vi "Login.vi"() -> ()   [LabVIEW 2020]
uses:
  Global1.vi
panel:
  in  "联机模式":enum16{"单机", "追溯"}(ring)
  in  "密码":string
  in  "账号":string
  in  "确定":bool
  # "芯轴分总成磨合台"
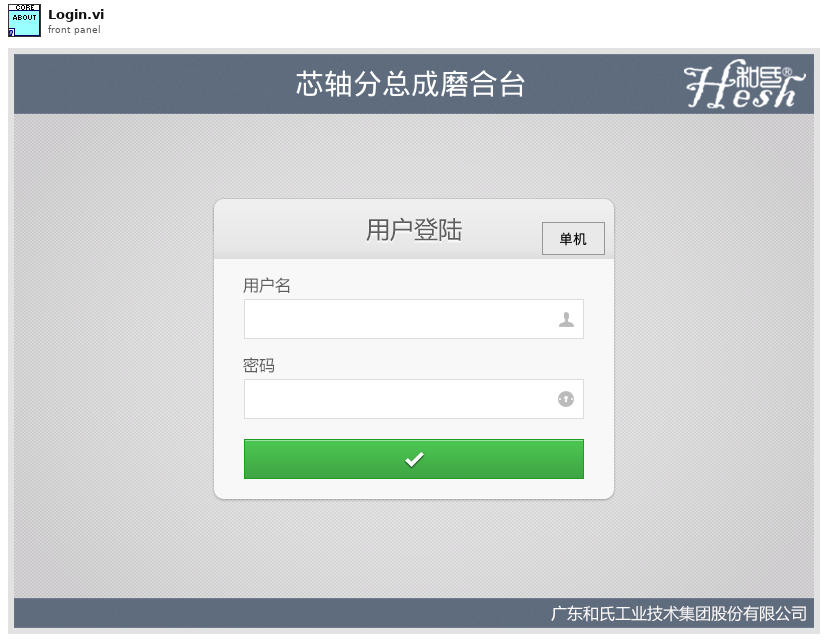
[diagram p1: front panel]
types:
  T1 = enum32{"Invalid", "Standard", "Closed", "Hidden", "Minimized", "Maximized"}
  T2 = enum8{"Enabled", "Disabled", "Disabled and Grayed Out"}
  T3 = cluster{"data[0]":string, "data[1]":string, "data[2]":string, "data[3]":string}
  T4 = typedef "eventvkey.ctl" = enum16{"ASCII", "Enter", "Return", "Shift", "Ctrl", "Alt", "Cmd", "Opt", "Caps", "NumLock", "Clear", "Break", "Up", "Down", "Left", "Right", "Insert", "Delete", "Home", "End", "PageUp", "PageDown", "Escape", "Help", "Pause", "ScrollLock", "F1", "F2", "F3", "F4", "F5", "F6", "F7", "F8", "F9", "F10", "F11", "F12", "F13", "F14", "F15", "F16", "F17", "F18", "F19", "F20", "F21", "F22", "F23", "F24", "Play", "VolumeUp", "VolumeDown", "Mute", "Two Byte Char"}
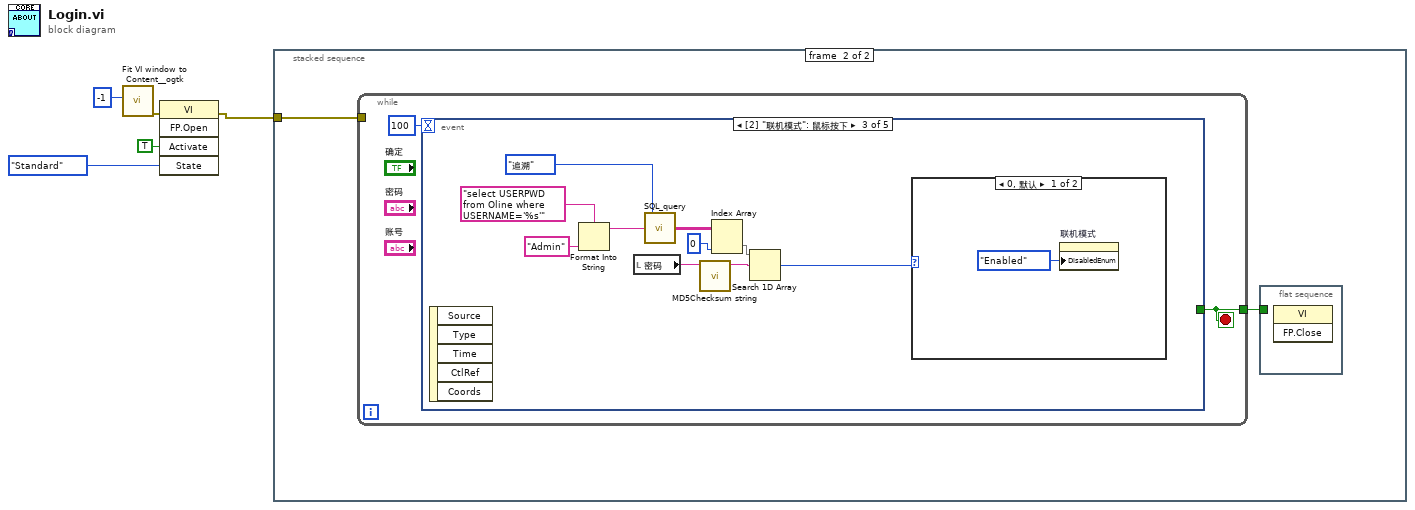
[diagram p0: block diagram]
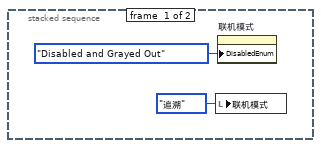
[diagram p2: hidden frame]
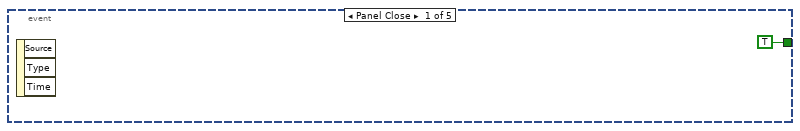
[diagram p3: hidden frame]
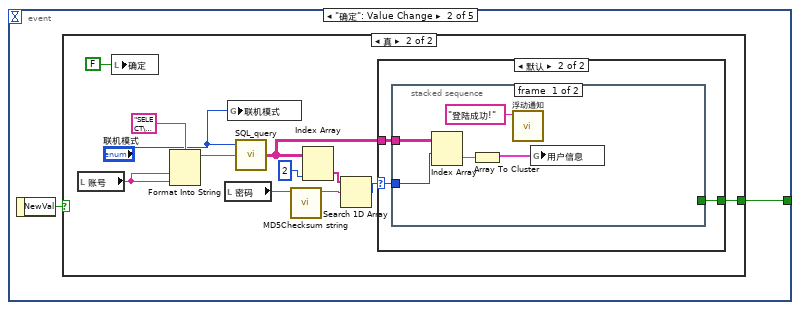
[diagram p4: hidden frame]
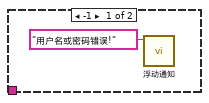
[diagram p6: hidden frame]
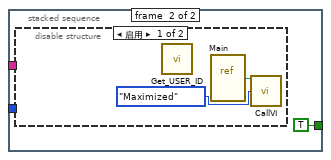
[diagram p7: hidden frame]
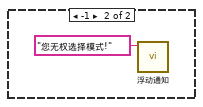
[diagram p9: hidden frame]
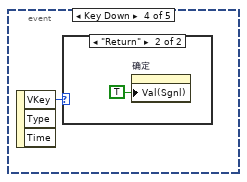
[diagram p10: hidden frame]
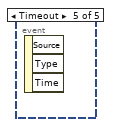
[diagram p12: hidden frame]
diagram:
  n1 = call <userlib>:"Fit VI window to Content__ogtk.vi"("border spacing (2 px)"=-1) -> ("error out"=w2:errorcluster)  [unwired: 5 in, 1 out]
  n2 = invoke class="VI" method="FP.Open"(error in=w2, "Activate"=TRUE ("Activate?"), "State"=T1."Standard") -> (error out=w1:errorcluster)  [unwired: 2 in, 4 out]
  n3 = stacked-sequence {
    tunnel: w1 -> [_ w8]
    frame #0 {
      n4 = local write "联机模式"(enum16{"单机", "追溯"}."追溯" ("联机模式")) -> ()
      n5 = property on="联机模式" class="Enum (严格)"("DisabledEnum"=T2."Disabled and Grayed Out" ("禁用")) -> ()  [unwired: 2 in, 2 out]
    }
    frame #1 {
      n6 = while {
        tunnel: [w11] -> w9
        tunnel: w8 -> [_]
        stop <- w11 stop-if-true
        n7 = event shown="[2] \"联机模式\": 鼠标按下" {
          selector: _ -> [_ _ _ _ _]
          dyn-events: _ -> [_ _ _ _ _]
          timeout: 100 -> [_ _ _ _ _]
          tunnel: [TRUE w13 _ _ _] -> w11
          event Panel Close {
            n8 = event-data() -> ()  [unwired: 4 out]
          }
          event "确定": Value Change {
            n9 = event-data() -> ("NewVal"=w14:bool)  [unwired: 1 out]
            n10 = case shown="真" w14 {
              tunnel: [_ w17] -> w13
              frame False {
              }
              frame True {
                n11 = local read "账号"() -> (w23:string)
                n12 = local write "确定"(FALSE ("确定")) -> ()
                n13 = Format Into String(format string="SELECT\ndbo.[User].USER_EMPLOYEE_ID,\ndbo.[User].USER_NAME,\ndbo.[User].USER_PASSWD,\ndbo.[User].USER_PERMIT\n\nFROM\ndbo.[User]\nWHERE\ndbo.[User].USER_NAME = '%s' \nOR\ndbo.[User].USER_EMPLOYEE_ID = '%s'\n" ("格式字符串"), w23, w23) -> (resulting string=w20:string)  [unwired: 2 in, 1 out]
                n14 = local read "密码"() -> (w24:string)
                n15 = global write "Global1.vi" "联机模式"("联机模式") -> ()
                n16 = call "SQL_query.vi"("SQL query"=w20, "联机模式"="联机模式") -> ("data"=w18:string[][])  [unwired: 1 in, 2 out]
                n17 = call <vilib>:"MD5Checksum string.vi"("Message String"=w24) -> ("MD5 message-digest"=w25:string)  [unwired: 10 in]
                n18 = Index Array(array=w18, index (col)=2 ("禁用的索引 (列)")) -> (element=w22:string[])  [unwired: 1 in]
                n19 = Search 1D Array(1D array=w22, element=w25) -> (index of element=w19:i32)  [unwired: 1 in]
                n20 = case shown="默认" w19 {
                  selector: w19 -> [_ w29]
                  tunnel: w18 -> [_ w30]
                  tunnel: [_ w28] -> w17
                  frame -1 {
                    n21 = call "浮动通知.vi"("通知内容"="用户名或密码错误!") -> ()  [unwired: 11 in]
                  }
                  frame Default {
                    n22 = stacked-sequence {
                      tunnel: w30 -> [w35 _]
                      tunnel: w29 -> [w34 _]
                      tunnel: [_ TRUE] -> w28
                      frame #0 {
                        n23 = Index Array(array=w35, index (row)=w34) -> (element=w32:string[])  [unwired: 1 in]
                        n24 = Array To Cluster(array=w32) -> (cluster=w31:T3)
                        n25 = call "浮动通知.vi"("通知内容"="登陆成功!") -> ()  [unwired: 11 in]
                        n26 = global write "Global1.vi" "用户信息"(w31) -> ()
                      }
                      frame #1 {
                        n27 = disable-structure shown="启用" {
                          frame Enabled {
                            n28 = call "Get_USER_ID.vi"() -> ()  [unwired: 10 in, 2 out]
                            n29 = vi-ref "Main.vi"() -> (w38:refnum<vi>)
                            n30 = call "CallVI.vi"("VI引用"=w38, "状态"=T1."Maximized") -> ()  [unwired: 11 in, 3 out]
                          }
                          frame Disabled {
                          }
                        }
                      }
                    }
                  }
                }
              }
            }
          }
          event "联机模式": Mouse Down {
            n31 = event-data() -> ()  [unwired: 6 out]
            n32 = Format Into String(format string="select USERPWD from Oline where USERNAME='%s'" ("格式字符串"), "Admin" ("输入 1")) -> (resulting string=w45:string)  [unwired: 2 in, 1 out]
            n33 = local read "密码"() -> (w47:string)
            n34 = call "SQL_query.vi"("SQL query"=w45, "联机模式"=enum16{"单机", "追溯"}."追溯") -> ("data"=w44:string[][])  [unwired: 1 in, 2 out]
            n35 = call <vilib>:"MD5Checksum string.vi"("Message String"=w47) -> ("MD5 message-digest"=w48:string)  [unwired: 10 in]
            n36 = Index Array(array=w44, index (col)=0 ("禁用的索引 (列)")) -> (element=w46:string[])  [unwired: 1 in]
            n37 = Search 1D Array(1D array=w46, element=w48) -> (index of element=w41:i32)  [unwired: 1 in]
            n38 = case shown="0, 默认" w41 {
              frame 0, Default {
                n39 = property on="联机模式" class="Enum (严格)"("DisabledEnum"=T2."Enabled" ("禁用")) -> ()  [unwired: 2 in, 2 out]
              }
              frame -1 {
                n40 = call "浮动通知.vi"("通知内容"="您无权选择模式!") -> ()  [unwired: 11 in]
              }
            }
          }
          event Key Down {
            n41 = event-data() -> ("VKey"=w51:T4)  [unwired: 3 out]
            n42 = case shown="\"Return\"" w51 {
              frame Default {
              }
              frame "Return" {
                n43 = property on="确定" class="Bool (严格)"("Val(Sgnl)"=TRUE ("值(信号)")) -> ()  [unwired: 2 in, 2 out]
              }
            }
          }
          event Timeout {
            n44 = event-data() -> ()  [unwired: 4 out]
          }
        }
      }
      n45 = flat-sequence {
        tunnel: w9 -> [_]
        frame #0 {
          n46 = invoke class="VI" method="FP.Close"() -> ()  [unwired: 3 in, 3 out]
        }
      }
    }
  }
